vi "Configure Tuner.vi"(7 "Tuner Gain Mode (0: auto)":u16(ring) items=["Automatic", "Manual"], 8 "error in (no error)":errorcluster, 9 "Bandwidth (Hz) (0: auto)":u32, 10 "Gain":i32, 11 "device handle in":T1) -> (0 "error out":errorcluster, 3 "device handle out":T1)   [LabVIEW 2019, in "RTL-SDR.lvlib"]
uses:
  RTL-SDR.lvlib
  Controls/Device Handle.ctl
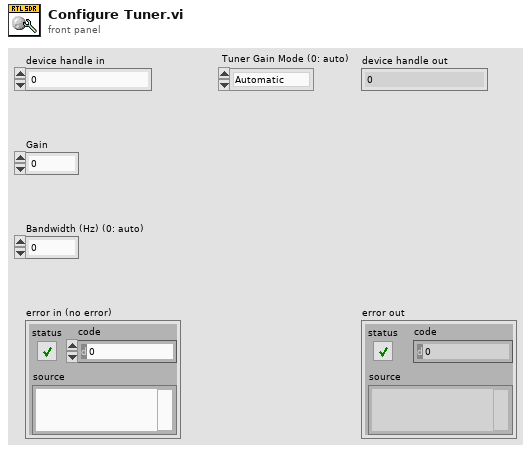
[diagram p1: front panel]
types:
  T1 = typedef "RTL-SDR.lvlib/Device Handle.ctl" = u64
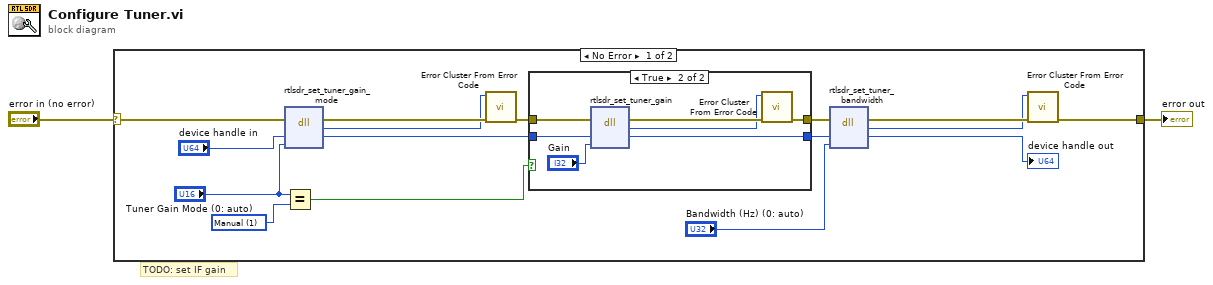
[diagram p0: block diagram]
diagram:
  # "TODO: set IF gain"
  n1 = case shown="No Error" "error in (no error)" {
    selector: "error in (no error)" -> [w18 w28]
    tunnel: [w4 w28] -> w2
    frame No Error {
      w10 = u16 1 items=["Automatic", "Manual"] ("Tuner Gain Mode 2")
      n2 = dll-call lib="usr/local/Cellar/librtlsdr/0.6.0/bin/rtl_sdr" fn="rtlsdr_set_tuner_gain_mode"(error in=w18, "dev"="device handle in", "manual"="Tuner Gain Mode (0: auto)") -> (error out=w17:errorcluster, "return type"=w13:i32, "dev"=w15:u64)  [unwired: 3 in, 1 out]
      n3 = Equal?(x="Tuner Gain Mode (0: auto)", y=w10) -> (x = y?=w12:bool)
      n4 = call <vilib>:"Error Cluster From Error Code.vi"("error in (no error)"=w17, "error code (0)"=w13) -> ("error out"=w14:errorcluster)  [unwired: 7 in]
      n5 = case shown="True" w12 {
        tunnel: [w20 w26] -> w9
        tunnel: w15 -> [w19 w24]
        tunnel: w14 -> [w20 w23]
        tunnel: [w19 w21] -> w7
        frame False {
        }
        frame True {
          n6 = dll-call lib="usr/local/Cellar/librtlsdr/0.6.0/bin/rtl_sdr" fn="rtlsdr_set_tuner_gain"(error in=w23, "dev"=w24, "gain"="Gain") -> (error out=w27:errorcluster, "return type"=w25:i32, "dev"=w21:u64)  [unwired: 3 in, 1 out]
          n7 = call <vilib>:"Error Cluster From Error Code.vi"("error in (no error)"=w27, "error code (0)"=w25) -> ("error out"=w26:errorcluster)  [unwired: 7 in]
        }
      }
      n8 = dll-call lib="usr/local/Cellar/librtlsdr/0.6.0/bin/rtl_sdr" fn="rtlsdr_set_tuner_bandwidth"(error in=w9, "dev"=w7, "bw"="Bandwidth (Hz) (0: auto)") -> (error out=w8:errorcluster, "return type"=w3:i32, "dev"=→"device handle out":u64)  [unwired: 3 in, 1 out]
      n9 = call <vilib>:"Error Cluster From Error Code.vi"("error in (no error)"=w8, "error code (0)"=w3) -> ("error out"=w4:errorcluster)  [unwired: 7 in]
    }
    frame Error {
    }
  }
  "error out" <- w2
